vi "Errors_Main.vi"(8 "error in":errorcluster, 11 "QRD":T1) -> (0 "error out":errorcluster)   [LabVIEW 2025]
uses:
  Controls/Queues-Refs-Data.ctl
  Builds/Queue Wrappers.lvlibp/Q Packet.ctl
  Controls/Local Data_Errors.ctl
  Controls/Error Packet.ctl
  Builds/Queue Wrappers.lvlibp
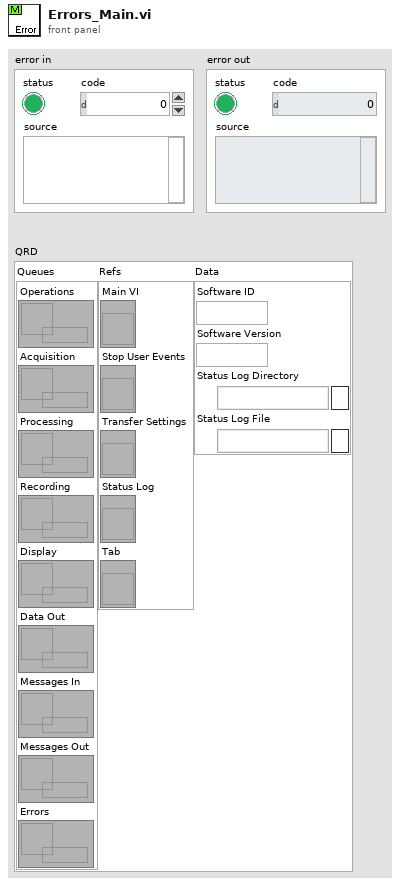
[diagram p1: front panel]
types:
  T1 = typedef "Queues-Refs-Data.ctl" = cluster{"Queues":cluster{"Operations":refnum<queue>, "Acquisition":refnum<queue>, "Processing":refnum<queue>, "Recording":refnum<queue>, "Display":refnum<queue>, "Data Out":refnum<queue>, "Messages In":refnum<queue>, "Messages Out":refnum<queue>, "Errors":refnum<queue>}, "Refs":cluster{"Main VI":refnum<vi>, "Stop User Events":refnum<vi>, "Transfer Settings":refnum<vi>, "Status Log":refnum<vi>, "Tab":refnum<vi>}, "Data":cluster{"Software ID":string, "Software Version":string, "Status Log Directory":path, "Status Log File":path}}
  T2 = typedef "Local Data_Errors.ctl" = cluster{"Loop ID":string}
  T3 = typedef "Error Packet.ctl" = cluster{"Time Stamp":timestamp, "Source":string, "Error":errorcluster}
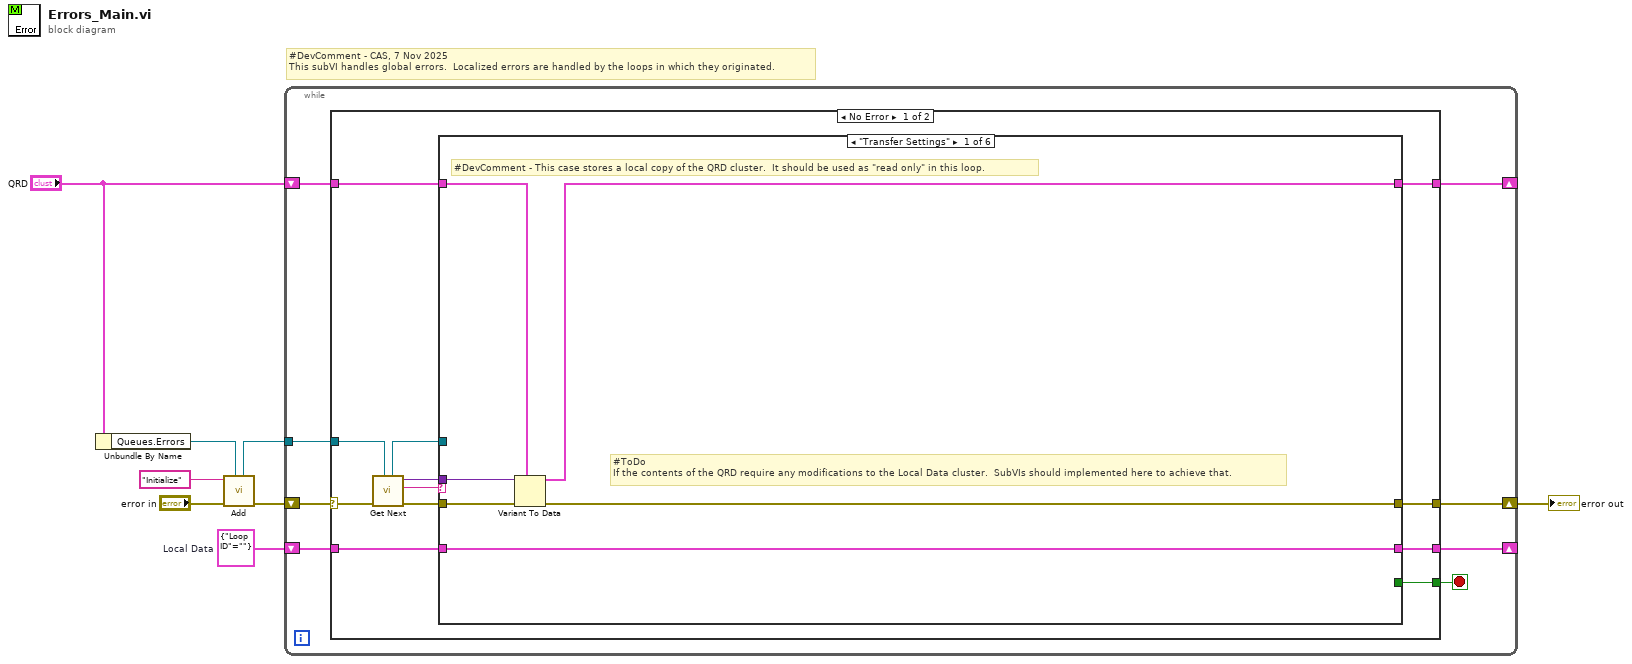
[diagram p0: block diagram]
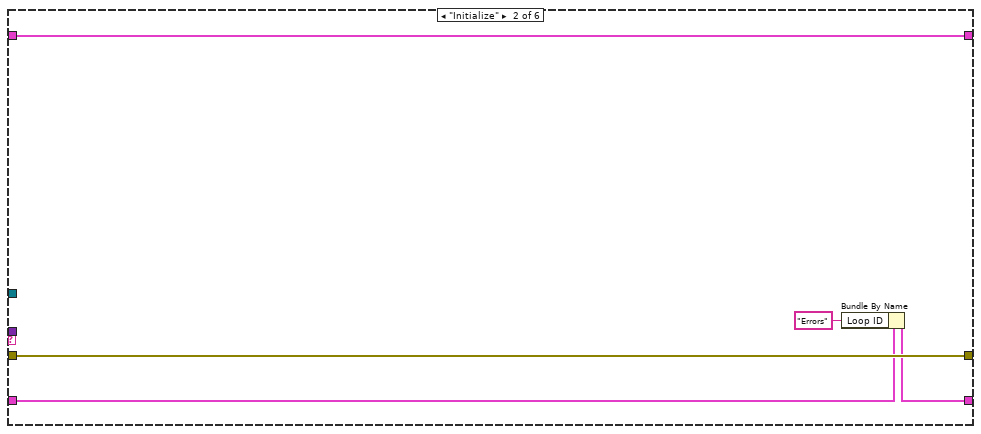
[diagram p2: hidden frame]
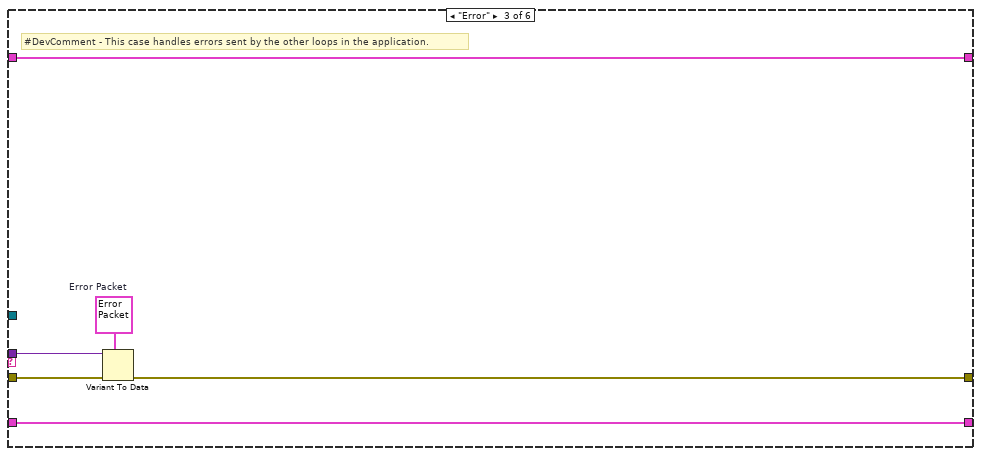
[diagram p3: hidden frame]
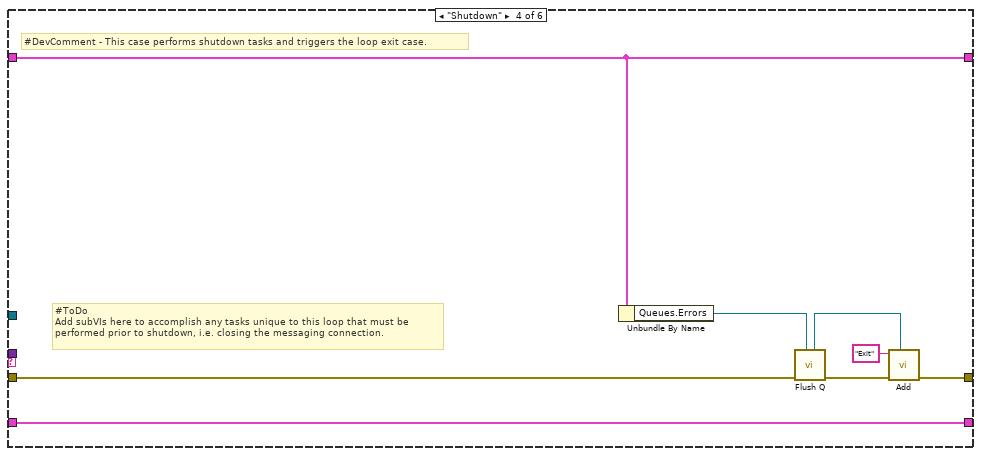
[diagram p4: hidden frame]
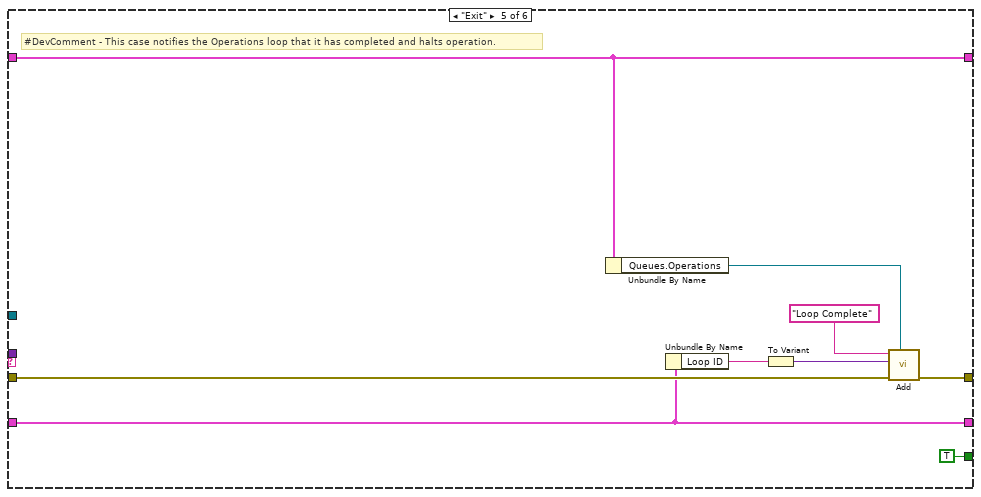
[diagram p5: hidden frame]
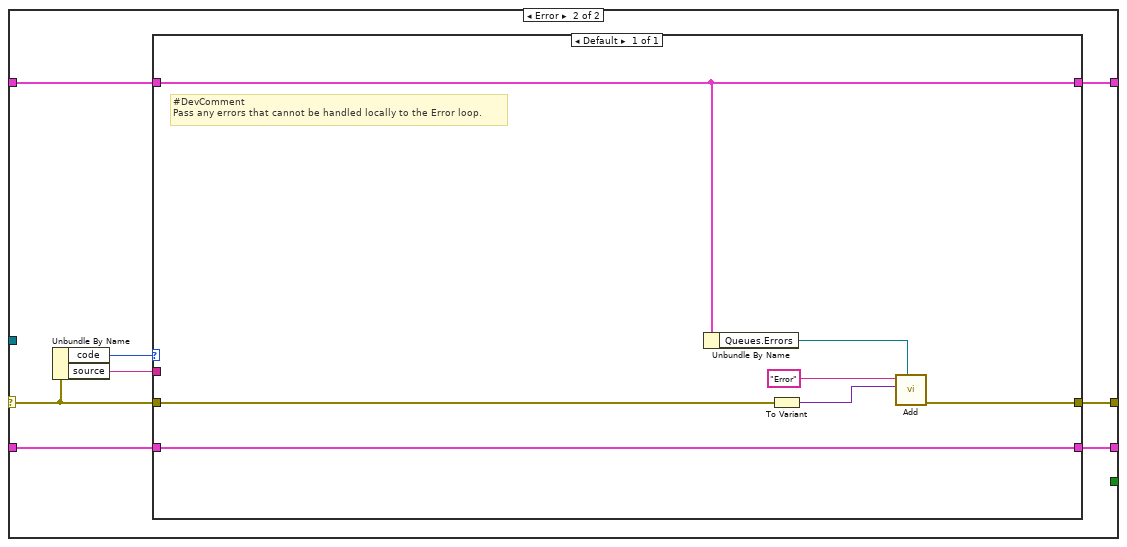
[diagram p7: hidden frame]
diagram:
  w6 = T2 {"Loop ID"=""}  # Local Data
  # "#DevComment - CAS, 7 Nov 2025\nThis subVI handles global errors.  Localized errors are handled by the loops in which they originated."
  n1 = Unbundle By Name("QRD") -> ("Queues.Errors"=w3:refnum<queue>)
  n2 = call "Add.vi"("Q Ref In"=w3, "error in"="error in", "Packet ID"="Initialize") -> ("error out"=w4:errorcluster, "Q Ref Out"=w2:refnum<queue>)  [unwired: 5 in, 2 out]
  n3 = while {
    shift-right: [w15] -> _
    shift-left: "QRD" -> [w16]
    shift-right: [w13] -> w8
    shift-left: w4 -> [w14]
    tunnel: w2 -> [w12]
    shift-right: [w9] -> _
    shift-left: w6 -> [w11]
    stop <- w10 stop-if-true
    n4 = case shown="No Error" w14 {
      selector: w14 -> [w28 w70]
      tunnel: w16 -> [w25 w67]
      tunnel: [w26 w68] -> w15
      tunnel: [w23 w69] -> w13
      tunnel: w12 -> [w27 _]
      tunnel: w11 -> [w19 w71]
      tunnel: [w18 w66] -> w9
      tunnel: [w17 _] -> w10
      frame No Error {
        n5 = call "Get Next.vi"("Q Ref In"=w27, "error in"=w28) -> ("error out"=w24:errorcluster, "Packet ID"=w20:string, "Payload"=w21:variant, "Q Ref Out"=w22:refnum<queue>)  [unwired: 6 in]
        n6 = case shown="\"Transfer Settings\"" w20 {
          tunnel: [w30 w38 w40 w53 w62 w65] -> w26
          tunnel: w25 -> [w32 w38 w40 w53 w62 w65]
          tunnel: w24 -> [w34 w39 w45 w50 w59 w64]
          tunnel: [w31 w39 w42 w52 w61 w64] -> w23
          tunnel: w22 -> [_ _ _ _ _ _]
          tunnel: w21 -> [w33 _ w44 _ _ _]
          tunnel: w19 -> [w29 w36 w41 w46 w57 w63]
          tunnel: [w29 w37 w41 w46 w57 w63] -> w18
          tunnel: [_ _ _ _ TRUE _] -> w17
          frame "Transfer Settings" {
            # "#ToDo\nIf the contents of the QRD require any modifications to the Local Data cluster.  SubVIs should implemented here to achieve that."
            # "#DevComment - This case stores a local copy of the QRD cluster.  It should be used as \"read only\" in this loop."
            n7 = Variant To Data(error in=w34, type=w32, Variant=w33) -> (data=w30:T1, error out=w31:errorcluster)
          }
          frame "Initialize" {
            n8 = Bundle By Name(cluster=w36, "Loop ID"="Errors") -> (w37:T2)
          }
          frame "Error" {
            w43 = T3 {"Time Stamp"=timestamp(0 s since 1904-01-01), "Source"="", "Error"={"status"=FALSE, "code"=0, "source"=""}}  # Error Packet
            # "#DevComment - This case handles errors sent by the other loops in the application."
            n9 = Variant To Data(error in=w45, type=w43, Variant=w44) -> (error out=w42:errorcluster)  [unwired: 1 out]
          }
          frame "Shutdown" {
            # "#ToDo\nAdd subVIs here to accomplish any tasks unique to this loop that must be\nperformed prior to shutdown, i.e. closing the messaging connection."
            # "#DevComment - This case performs shutdown tasks and triggers the loop exit case."
            n10 = Unbundle By Name(w53) -> ("Queues.Errors"=w48:refnum<queue>)
            n11 = call "Flush Q.vi"("Q Ref In"=w48, "error in"=w50) -> ("error out"=w49:errorcluster, "Q Ref Out"=w47:refnum<queue>)  [unwired: 8 in]
            n12 = call "Add.vi"("Q Ref In"=w47, "error in"=w49, "Packet ID"="Exit") -> ("error out"=w52:errorcluster)  [unwired: 5 in, 3 out]
          }
          frame "Exit" {
            # "#DevComment - This case notifies the Operations loop that it has completed and halts operation."
            n13 = Unbundle By Name(w62) -> ("Queues.Operations"=w58:refnum<queue>)
            n14 = Unbundle By Name(w57) -> ("Loop ID"=w56:string)
            n15 = To Variant(anything=w56) -> (Variant=w55:variant)
            n16 = call "Add.vi"("Q Ref In"=w58, "error in"=w59, "Payload"=w55, "Packet ID"="Loop Complete") -> ("error out"=w61:errorcluster)  [unwired: 4 in, 3 out]
          }
          frame Default {
          }
        }
      }
      frame Error {
        n17 = Unbundle By Name(w70) -> ("code"=w73:i32, "source"=w72:string)
        n18 = case shown="Default" w73 {
          tunnel: w72 -> [_]
          tunnel: w71 -> [w80]
          tunnel: [w80] -> w66
          tunnel: w70 -> [w75]
          tunnel: [w77] -> w69
          tunnel: [w76] -> w68
          tunnel: w67 -> [w76]
          frame Default {
            # "#DevComment\nPass any errors that cannot be handled locally to the Error loop."
            n19 = Unbundle By Name(w76) -> ("Queues.Errors"=w78:refnum<queue>)
            n20 = To Variant(anything=w75) -> (Variant=w74:variant)
            n21 = call "Add.vi"("Q Ref In"=w78, "Payload"=w74, "Packet ID"="Error") -> ("error out"=w77:errorcluster)  [unwired: 5 in, 3 out]
          }
        }
      }
    }
  }
  "error out" <- w8
